vi "FTW-Request-WriteResponse.vi"(0 "FTW Incoming Request":refnum<class "FTW-Request.lvclass">, 5 "Response Header":string, 7 "Response Body":string, 11 "error in":errorcluster) -> (4 "FTW Incoming Request out":refnum<class "FTW-Request.lvclass">, 15 "error out":errorcluster)   [LabVIEW 2013, in "FTW-Actor.lvlib" / "FTW-Request.lvclass"]
uses:
  FTW-Request.lvclass
  FTW-Request.lvclass/FTW-Request.ctl
  Core/src/JSON/FTW-JSON.lvclass
panel:
  # "Inputs"
  # "Outputs"
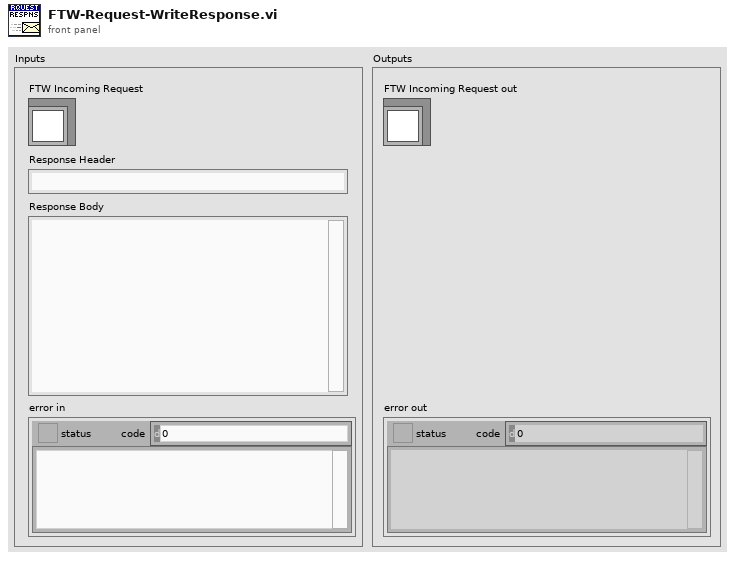
[diagram p1: front panel]
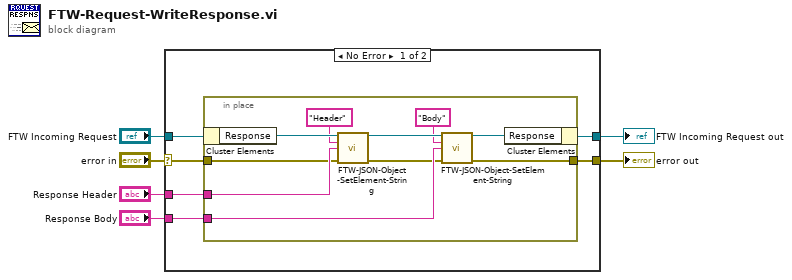
[diagram p0: block diagram]
diagram:
  n1 = case shown="No Error" "error in" {
    selector: "error in" -> [w8 w23]
    tunnel: [w7 w23] -> w5
    tunnel: [w11 w24] -> w4
    tunnel: "FTW Incoming Request" -> [w12 w24]
    tunnel: "Response Header" -> [w10 _]
    tunnel: "Response Body" -> [w9 _]
    frame No Error {
      n2 = in-place {
        in-place-border: w10 -> [w18]
        in-place-border: w9 -> [w17]
        in-place-border: w8 -> [w15]
        in-place-border: [w13] -> w7
        n3 = in-place-cluster #1(w12) -> ("Response"=w22:refnum<class "FTW-JSON.lvclass">)
        n4 = call "FTW-JSON-Object-SetElement-String.vi"("JSON Object"=w22, "Key"="Header", "Value"=w18, "error in"=w15) -> ("JSON Object out"=w21:refnum<class "FTW-JSON.lvclass">, "error out"=w14:errorcluster)  [unwired: 10 in]
        n5 = call "FTW-JSON-Object-SetElement-String.vi"("JSON Object"=w21, "Key"="Body", "Value"=w17, "error in"=w14) -> ("JSON Object out"=w20:refnum<class "FTW-JSON.lvclass">, "error out"=w13:errorcluster)  [unwired: 10 in]
        n6 = in-place-cluster #1("Response"=w20) -> (w11:refnum<class "FTW-Request.lvclass">)
      }
    }
    frame Error {
    }
  }
  "error out" <- w5
  "FTW Incoming Request out" <- w4
